vi "Delete.vi"(7 "Average Splitter?":bool, 8 "error in":errorcluster caption="错误输入（无错误）", 10 "Data":variant, 11 "PanelRootNode 输入":refnum<class "PanelRootNode.lvclass"> caption="DNL_LabVIEW Object in") -> (0 "error out":errorcluster caption="错误输出", 3 "PanelRootNode 输出":refnum<class "PanelRootNode.lvclass"> caption="DNL_LabVIEW Object out")   [LabVIEW 2016, in "PanelRootNode.lvclass"]
uses:
  PanelRootNode.lvclass
  PanelObject/PanelObject.lvclass
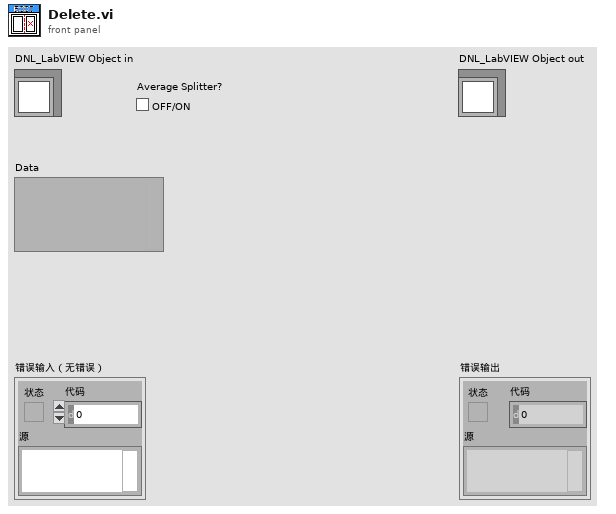
[diagram p1: front panel]
types:
  T1 = cluster{"Node*":refnum<data-value>, "AbortVI":bool}
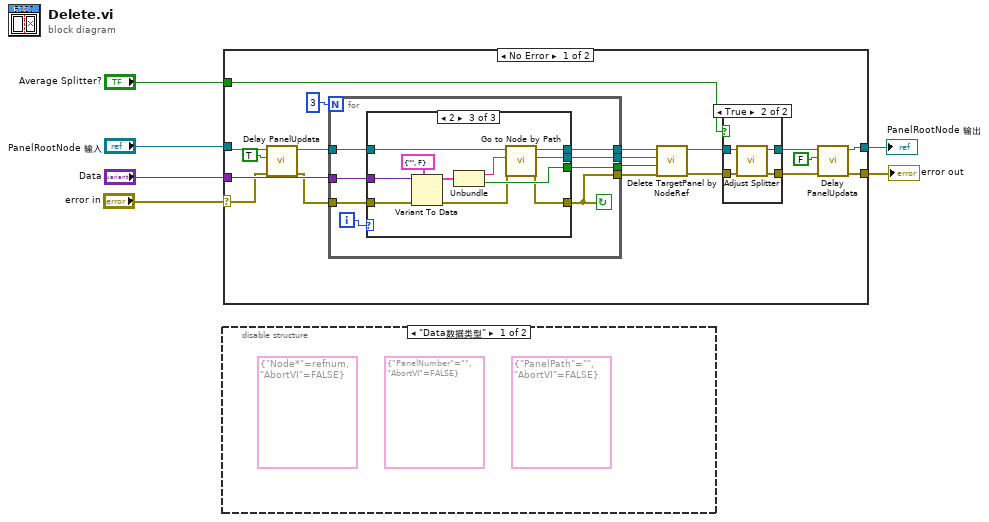
[diagram p0: block diagram]
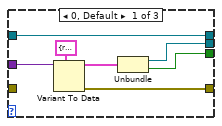
[diagram p4: hidden frame]
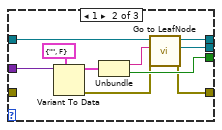
[diagram p5: hidden frame]
diagram:
  n1 = disable-structure shown="\"Data数据类型\"" {
    frame condition #0 {
      (unwired) cluster{"PanelPath":string, "AbortVI":bool} {"PanelPath"="", "AbortVI"=FALSE}
      (unwired) cluster{"PanelNumber":string, "AbortVI":bool} {"PanelNumber"="", "AbortVI"=FALSE}
      (unwired) T1 {"Node*"=refnum, "AbortVI"=FALSE}
    }
    frame condition #1 (active) {
    }
  }
  n2 = case shown="No Error" "error in" {
    selector: "error in" -> [w17 w69]
    tunnel: [w14 w69] -> w5
    tunnel: [w13 w68] -> w3
    tunnel: "PanelRootNode 输入" -> [w19 w68]
    tunnel: "Data" -> [w24 _]
    tunnel: "Average Splitter?" -> [w7 _]
    frame No Error {
      n3 = call "Delay PanelUpdata.vi"("error in"=w17, "延迟前面板更新"=TRUE, "PanelRootNode 输入"=w19) -> ("error out"=w16:errorcluster, "PanelRootNode 输出"=w18:refnum<class "PanelRootNode.lvclass">)  [unwired: 7 in]
      n4 = for {
        N: 3 -> [_]
        tunnel: [w38] -> w23
        tunnel: [w37] -> w21
        tunnel: w18 -> [w36]
        tunnel: [w35] -> w20
        tunnel: [w34] -> w22
        tunnel: w24 -> [w33]
        tunnel: w16 -> [w32]
        i -> [w39]
        stop <- w34 continue-if-true
        n5 = case shown="2" w39 {
          tunnel: [w46 w56 w67] -> w35
          tunnel: [w45 w52 w63] -> w37
          tunnel: [w42 w54 w65] -> w38
          tunnel: [w43 w51 w62] -> w34
          tunnel: w36 -> [w42 w49 w61]
          tunnel: w33 -> [w41 w48 w59]
          tunnel: w32 -> [_ _ w57]
          frame 0, Default {
            n6 = Variant To Data(type=T1 {"Node*"=refnum, "AbortVI"=FALSE}, Variant=w41) -> (data=w44:T1, error out=w43:errorcluster)  [unwired: 1 in]
            n7 = Unbundle(w44) -> ("Node*"=w45:refnum<data-value>, "AbortVI"=w46:bool)
          }
          frame 1 {
            n8 = Variant To Data(type=cluster{"PanelNumber":string, "AbortVI":bool} {"PanelNumber"="", "AbortVI"=FALSE}, Variant=w48) -> (data=w55:cluster{"PanelNumber":string, "AbortVI":bool}, error out=w50:errorcluster)  [unwired: 1 in]
            n9 = Unbundle(w55) -> ("PanelNumber"=w53:string, "AbortVI"=w56:bool)
            n10 = call-dynamic "Go to LeafNode.vi"("error in"=w50, "LeafNumber"=w53, "PanelRootNode 输入"=w49) -> ("error out"=w51:errorcluster, "Node*"=w52:refnum<data-value>, "PanelRootNode 输出"=w54:refnum<class "PanelRootNode.lvclass">)  [unwired: 5 in, 1 out]
          }
          frame 2 {
            n11 = Variant To Data(error in=w57, type=cluster{"PanelPath":string, "AbortVI":bool} {"PanelPath"="", "AbortVI"=FALSE}, Variant=w59) -> (data=w66:cluster{"PanelPath":string, "AbortVI":bool}, error out=w60:errorcluster)
            n12 = Unbundle(w66) -> ("PanelPath"=w64:string, "AbortVI"=w67:bool)
            n13 = call-dynamic "Go to Node by Path.vi"("error in"=w60, "NodePath"=w64, "PanelLinkNode 输入"=w61) -> ("error out"=w62:errorcluster, "Node*"=w63:refnum<data-value>, "PanelLinkNode 输出"=w65:refnum<class "PanelRootNode.lvclass">)  [unwired: 5 in, 1 out]
          }
        }
      }
      n14 = call-dynamic "Delete TargetPanel by NodeRef.vi"("error in"=w22, "Abort VI"=w20, "Node*"=w21, "PanelRootNode 输入"=w23) -> ("error out"=w10:errorcluster, "PanelRootNode 输出"=w11:refnum<class "PanelRootNode.lvclass">)  [unwired: 6 in]
      n15 = case shown="True" w7 {
        tunnel: w11 -> [w27 w31]
        tunnel: [w27 w30] -> w8
        tunnel: w10 -> [w26 w29]
        tunnel: [w26 w28] -> w9
        frame False {
        }
        frame True {
          n16 = call "Adjust Splitter.vi"("error in (no error)"=w29, "PanelRootNode 输入"=w31) -> ("error out"=w28:errorcluster, "PanelRootNode 输出"=w30:refnum<class "PanelRootNode.lvclass">)  [unwired: 8 in]
        }
      }
      n17 = call "Delay PanelUpdata.vi"("error in"=w9, "延迟前面板更新"=FALSE, "PanelRootNode 输入"=w8) -> ("error out"=w14:errorcluster, "PanelRootNode 输出"=w13:refnum<class "PanelRootNode.lvclass">)  [unwired: 7 in]
    }
    frame Error {
    }
  }
  "error out" <- w5
  "PanelRootNode 输出" <- w3
